vi "Controller Read FXP20.5.vi"(3 "error in (no error)":errorcluster, 5 "Variables":refnum<k21>[](array[refnum])) -> (0 "error out":errorcluster, 1 "Values":fxp<+/-,20,5>[](array[numeric]) format="%.17g")   [LabVIEW 2011, in "Controller VIs.lvlib"]
doc: "Reads a vector of fixed-Point <+/-,20,5> I/O variables."
uses:
  Controller VIs.lvlib
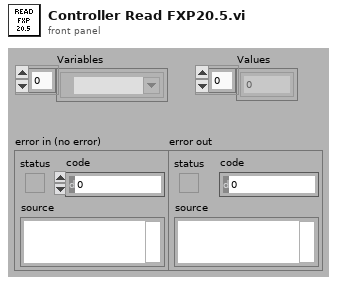
[diagram p1: front panel]
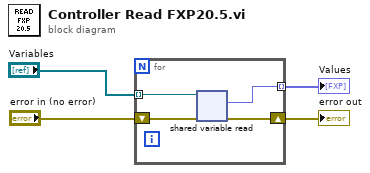
[diagram p0: block diagram]
diagram:
  n1 = for {
    tunnel: "Variables" -> [w8] mode=indexing
    tunnel: [w7] -> w2 mode=indexing
    shift-right: [w5] -> w3
    shift-left: "error in (no error)" -> [w6]
    n2 = shared-variable-read(w8, w6) -> (w5:errorcluster, w7:fxp<+/-,20,5>)  [unwired: 2 out]
  }
  "Values" <- w2
  "error out" <- w3
